vi "sendResponse.vi"(0 "Mockbus in":refnum<class "Mockbus.lvclass">, 5 "AllGood?":bool, 11 "error in (no error)":errorcluster) -> (4 "Mockbus out":refnum<class "Mockbus.lvclass">, 15 "error out":errorcluster)   [LabVIEW 2015, in "RTMockbus.lvlib" / "Mockbus.lvclass"]
uses:
  Mockbus.lvclass
  Mockbus.lvclass/Mockbus.ctl
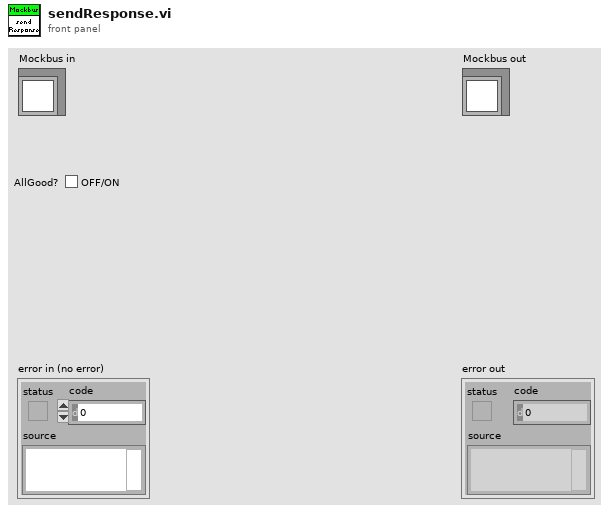
[diagram p1: front panel]
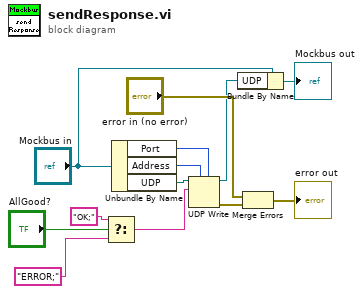
[diagram p0: block diagram]
diagram:
  n1 = Select(t="OK;", s="AllGood?", f="ERROR;") -> (s? t:f=w11:string)
  n2 = Unbundle By Name("Mockbus in") -> ("Port"=w2:u16, "Address"=w1:u32, "UDP"=w13:refnum<k16>)
  n3 = UDP Write(address=w1, port or service name=w2, connection ID=w13, data in=w11) -> (error out=w8:errorcluster, 3:w3:refnum<k16>)  [unwired: 2 in]
  n4 = Bundle By Name(cluster="Mockbus in", "UDP"=w3) -> (→"Mockbus out":refnum<class "Mockbus.lvclass">)
  n5 = Merge Errors("error in (no error)", w8) -> (→"error out":errorcluster)
